vi "milliGAT_standalone.vi"() -> ()   [LabVIEW 2017]
uses:
  <vilib>/Instr/_visa.llb/VISA Configure Serial Port (Instr).vi
panel:
  in  "flow control":u16(ring) items=["None"=0, "XON/XOFF"=1, "RTS/CTS"=2, "DTR/DSR"=4]
  in  "stop bits":u16(ring)=10 items=["1.0"=10, "1.5"=15, "2.0"=20]
  in  "parity":u16(ring) items=["None", "Odd", "Even", "Mark", "Space"]
  in  "data bits":u16=8 min=5 max=8 step=1
  in  "VISA resource name":refnum<visa-resource-name>="COM1"
  in  "baud rate":u32=9600
  out "Answer":string
  in  "Tell":bool
  in  "?":u16(ring) items=["Constant flowrate, 0.0005<n<167uL/s", "Maximum flowrate, 0.001<n<167 uL/s", "Dispense Set Volume, 0.001<n<1E15 uL", "Aspirate Set Volume, 0.001<n<1E15 uL", "Stop Pump"]
  out "bytes read 2":u32
  in  "User Input":i32
  in  "Stop":bool
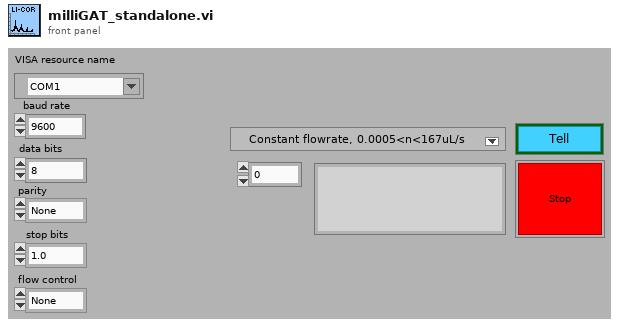
[diagram p1: front panel]
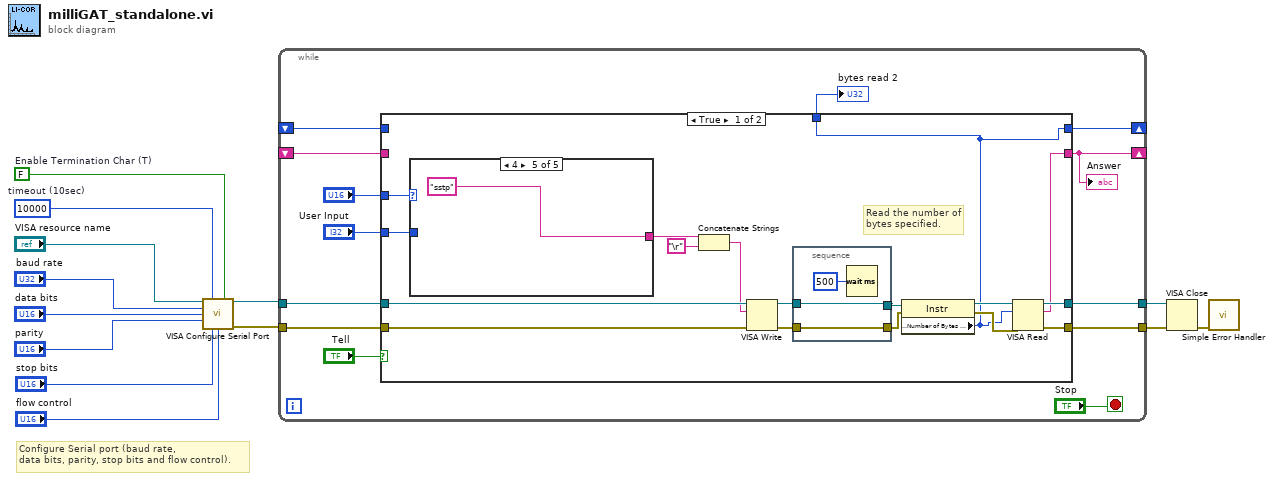
[diagram p0: block diagram]
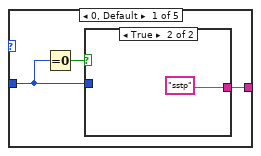
[diagram p2: hidden frame]
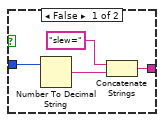
[diagram p3: hidden frame]
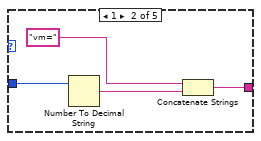
[diagram p4: hidden frame]
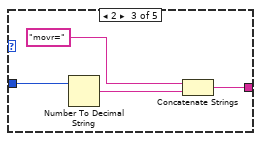
[diagram p5: hidden frame]
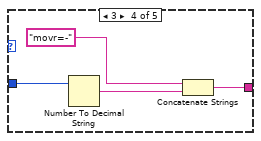
[diagram p6: hidden frame]
diagram:
  w6 = FALSE  # Enable Termination Char (T)
  w7 = u32 10000  # timeout (10sec)
  # "Configure Serial port (baud rate,\ndata bits, parity, stop bits and flow control)."
  n1 = call-poly "VISA Configure Serial Port"("VISA resource name"="VISA resource name", "timeout (10sec)"=w7, "Enable Termination\nChar (T)"=w6, "baud rate (9600)"="baud rate", "data bits (8)"="data bits", "parity (0:none)"="parity", "stop bits (10: 1 bit)"="stop bits", "flow control (0:none)"="flow control") -> ("VISA resource name out"=w2:refnum<visa-resource-name>, "error out"=w1:errorcluster)  [unwired: 6 in]
  n2 = while {
    tunnel: w2 -> [w25]
    tunnel: w1 -> [w24]
    tunnel: [w22] -> w12
    tunnel: [w21] -> w11
    shift-right: [w17] -> _
    shift-left: _ -> [w16]
    shift-right: [w15] -> _
    shift-left: _ -> [w14]
    stop <- "Stop" stop-if-true
    n3 = case shown="True" "Tell" {
      tunnel: w25 -> [w36 w69]
      tunnel: w24 -> [w35 w68]
      tunnel: [w33 w69] -> w22
      tunnel: [w32 w68] -> w21
      tunnel: [w28 w70] -> w23
      tunnel: "User Input" -> [w31 _]
      tunnel: "?" -> [w29 _]
      tunnel: [w27 w71] -> w17
      tunnel: w16 -> [_ w71]
      tunnel: [w28 w70] -> w15
      tunnel: w14 -> [_ w70]
      frame True {
        # "Read the number of bytes specified."
        n4 = case shown="4" w29 {
          tunnel: [w46 w55 w59 w63 "sstp"] -> w43
          tunnel: w31 -> [w44 w54 w58 w62 _]
          frame 0, Default {
            n5 = Equal To 0?(x=w44) -> (x = 0?=w45:bool)
            n6 = case shown="True" w45 {
              tunnel: [w50 "sstp"] -> w46
              tunnel: w44 -> [w49 _]
              frame False {
                n7 = Number To Decimal String(number=w49) -> (decimal integer string=w47:string)  [unwired: 1 in]
                n8 = Concatenate Strings("slew=", w47) -> (w50:string)
              }
              frame True {
              }
            }
          }
          frame 1 {
            n9 = Number To Decimal String(number=w54) -> (decimal integer string=w52:string)  [unwired: 1 in]
            n10 = Concatenate Strings("vm=", w52) -> (w55:string)
          }
          frame 2 {
            n11 = Number To Decimal String(number=w58) -> (decimal integer string=w56:string)  [unwired: 1 in]
            n12 = Concatenate Strings("movr=", w56) -> (w59:string)
          }
          frame 3 {
            n13 = Number To Decimal String(number=w62) -> (decimal integer string=w60:string)  [unwired: 1 in]
            n14 = Concatenate Strings("movr=-", w60) -> (w63:string)
          }
          frame 4 {
          }
        }
        n15 = Concatenate Strings(w43, "\r") -> (w34:string)
        n16 = VISA Write(VISA resource name=w36, write buffer=w34, error in (no error)=w35) -> (VISA resource name out=w42:refnum<visa-resource-name>, error out=w41:errorcluster)  [unwired: 1 out]
        n17 = stacked-sequence {
          tunnel: w42 -> [w67]
          tunnel: w41 -> [w66]
          tunnel: [w67] -> w38
          tunnel: [w66] -> w37
          frame #0 {
            n18 = Wait (ms)(milliseconds to wait=u32 500) -> ()  [unwired: 1 out]
          }
        }
        n19 = property class="Instr"(reference=w38, error in=w37) -> (reference out=w40:refnum<visa-resource-name>, error out=w39:errorcluster, "Serial Settings:Number of Bytes at Serial Port"=w28:u32)
        n20 = VISA Read(VISA resource name=w40, byte count=w28, error in (no error)=w39) -> (VISA resource name out=w33:refnum<visa-resource-name>, read buffer=w27:string, error out=w32:errorcluster)  [unwired: 1 out]
      }
      frame False {
      }
    }
    "bytes read 2" <- w23
    "Answer" <- w17
  }
  n21 = VISA Close(VISA resource name=w12, error in (no error)=w11) -> (error out=w13:errorcluster)
  n22 = call <vilib>:"Simple Error Handler.vi"("error in (no error)"=w13) -> ()  [unwired: 1 in, 8 out]
